vi "initialise camera.vi"(8 "error in (no error)":errorcluster, 11 "Cascade in":refnum<class "Cascade.lvclass">) -> (0 "error out":errorcluster, 3 "Cascade out":refnum<class "Cascade.lvclass">)   [LabVIEW 2012, in "Cascade.lvclass"]
uses:
  Cascade.lvclass
  Cascade.lvclass/Cascade.ctl
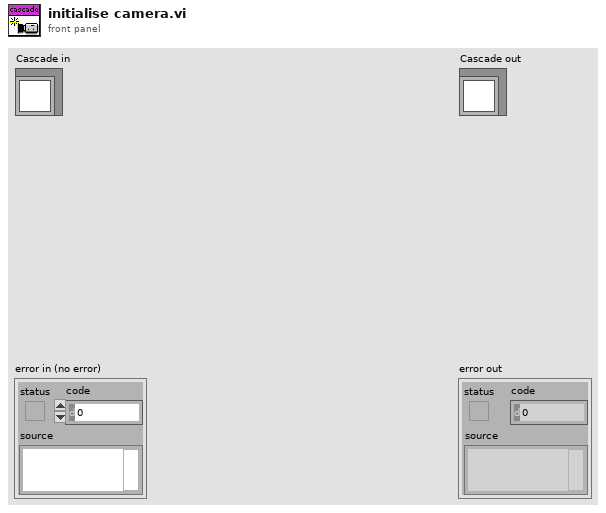
[diagram p1: front panel]
types:
  T1 = typedef "Cascade.lvclass/acquire flag.ctl" = u32
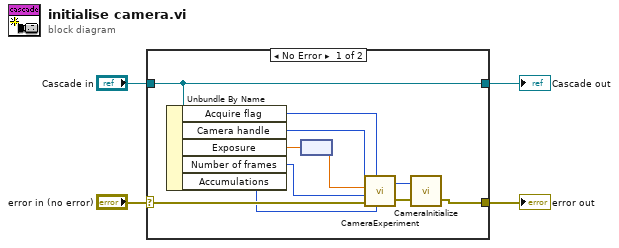
[diagram p0: block diagram]
diagram:
  n1 = case shown="No Error" "error in (no error)" {
    selector: "error in (no error)" -> [w13 w17]
    tunnel: [w12 w17] -> w3
    tunnel: [w11 w16] -> w1
    tunnel: "Cascade in" -> [w11 w16]
    frame No Error {
      n2 = Unbundle By Name(w11) -> ("Acquire flag"=w6:T1, "Camera handle"=w10:u32, "Exposure"=w9:dbl[unit], "Number of frames"=w7:u32, "Accumulations"=w5:u32)
      n3 = node(w9) -> (w8:dbl)
      n4 = call <userlib>:"CameraExperiment.vi"("Number of Accumulations"=w5, "Acquire / Focus Flag"=w6, "error in"=w13, "Number of Images"=w7, "Exposure (sec)"=w8, "Camera Handle"=w10) -> ("error out"=w15:errorcluster, "Camera Handle"=w14:u32)
      n5 = call <userlib>:"CameraInitialize.vi"("error in"=w15, "Camera Handle"=w14) -> ("error out"=w12:errorcluster)  [unwired: 1 out]
    }
    frame Error {
    }
  }
  "error out" <- w3
  "Cascade out" <- w1
